vi "16-ParseNumberOfSubPackets.vi"(11 "BITS in":bool[](array[boolean])) -> (2 "Number of Sub Packets":u32, 3 "BITS out":bool[](array[boolean]))   [LabVIEW 2019, in "16.lvlib"]
uses:
  16.lvlib
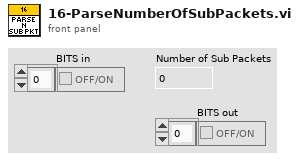
[diagram p1: front panel]
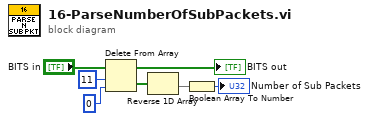
[diagram p0: block diagram]
diagram:
  n1 = Delete From Array(array="BITS in", length=11, index=0) -> (deleted portion=w5:bool[], array with subset deleted=→"BITS out":bool[])
  n2 = Reverse 1D Array(array=w5) -> (reversed array=w4:bool[])
  n3 = Boolean Array To Number(Boolean array=w4) -> (number=→"Number of Sub Packets":u32)
